vi "Write msg.vi"(8 "error in (no error)":errorcluster, 10 "msg":string, 11 "Message Step in":refnum<class "Message Step.lvclass">) -> (0 "error out":errorcluster, 3 "Message Step out":refnum<class "Message Step.lvclass">)   [LabVIEW 2017, in "Controller.lvlib" / "Message Step.lvclass"]
uses:
  Message Step.lvclass
  Message Step.lvclass/Message Step.ctl
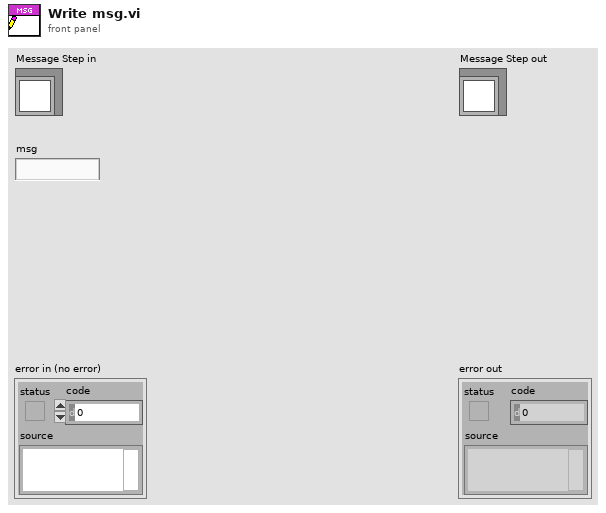
[diagram p1: front panel]
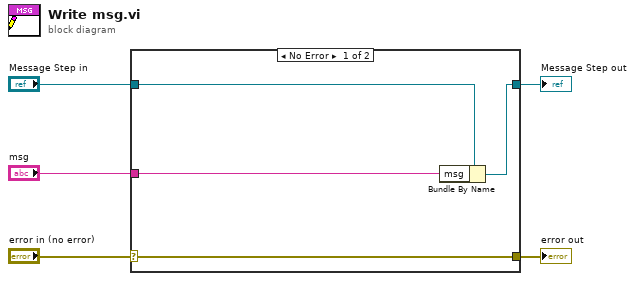
[diagram p0: block diagram]
diagram:
  n1 = case shown="No Error" "error in (no error)" {
    selector: "error in (no error)" -> [w9 w10]
    tunnel: [w9 w10] -> w4
    tunnel: [w7 w11] -> w2
    tunnel: "Message Step in" -> [w8 w11]
    tunnel: "msg" -> [w6 _]
    frame No Error {
      n2 = Bundle By Name(cluster=w8, "msg"=w6) -> (w7:refnum<class "Message Step.lvclass">)
    }
    frame Error {
    }
  }
  "error out" <- w4
  "Message Step out" <- w2
